vi "Tree Control - Update Symbols.vi"(8 "error in (no error)":errorcluster, 10 "route specification":string, 11 "tree refnum":refnum<vi>) -> (0 "error out":errorcluster, 3 "tree refnum out":refnum<vi>)   [LabVIEW 2025, in "Switch Executive Controller UI.lvlib"]
uses:
  Switch Executive Controller UI.lvlib
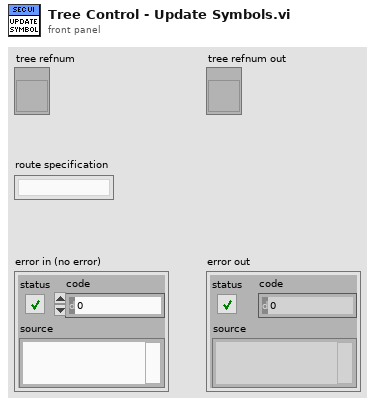
[diagram p1: front panel]
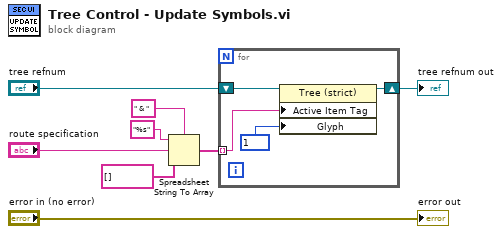
[diagram p0: block diagram]
diagram:
  n1 = Spreadsheet String To Array(delimiter (Tab)=" & ", format string="%s", spreadsheet string="route specification", array type (2D Dbl)=string[] []) -> (array=w1:string[])
  n2 = for {
    shift-right: [w12] -> w3
    shift-left: "tree refnum" -> [w11]
    tunnel: w1 -> [w10] mode=indexing
    n3 = property class="Tree (strict)"(reference=w11, "Active Item Tag"=w10, "Glyph"=1) -> (reference out=w12:refnum<vi>)  [unwired: 1 in, 1 out]
  }
  "tree refnum out" <- w3
  "error out" <- "error in (no error)"
